vi "QD_git.vi"(6 "Variant in":variant, 7 "Shift Pressed?":bool, 8 "error in (no error)":errorcluster, 10 "QD Combo Box Ref":refnum<vi>, 11 "QD Launch VI Ref":refnum<vi>) -> (0 "error out":errorcluster, 4 "Variant out":variant)   [LabVIEW 2020, in "AJ_QuickDrop_Git.lvlib"]
doc: "Write a 1-2 sentence description of the functionality of your plugin here. Replace the \"$\" below with the character you wish to assign as the default shortcut for this plugin. Do not add any text after the 'Default Shortcut' line below.\n\nDefault Shortcut - [$]"
uses:
  <resource>/dialog/QuickDrop/plugins/AJ_QD_Git/AJ_QuickDrop_Git.lvlib
panel:
  in  "Undo Name":string="Quick Drop Keyboard Shortcut"
  # "Do not change the connector pane of this VI.\n\nSee the block diagram for directions on how to use this template."
  # "Specify the name of the Undo transaction"
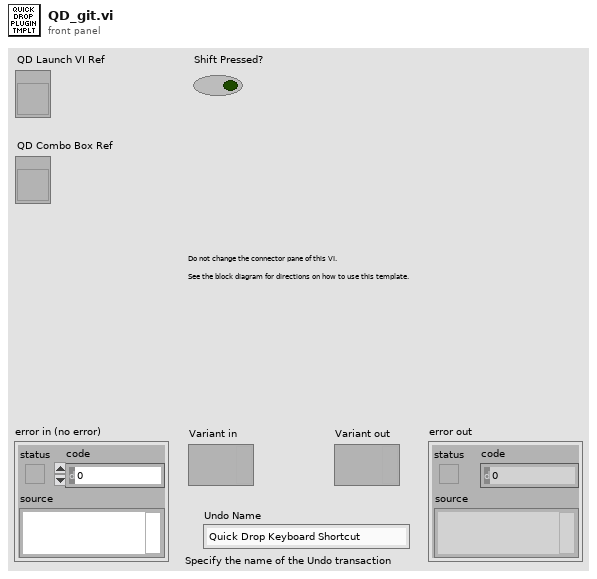
[diagram p1: front panel]
types:
  T1 = enum32{"Invalid", "Standard", "Closed", "Hidden", "Minimized", "Maximized"}
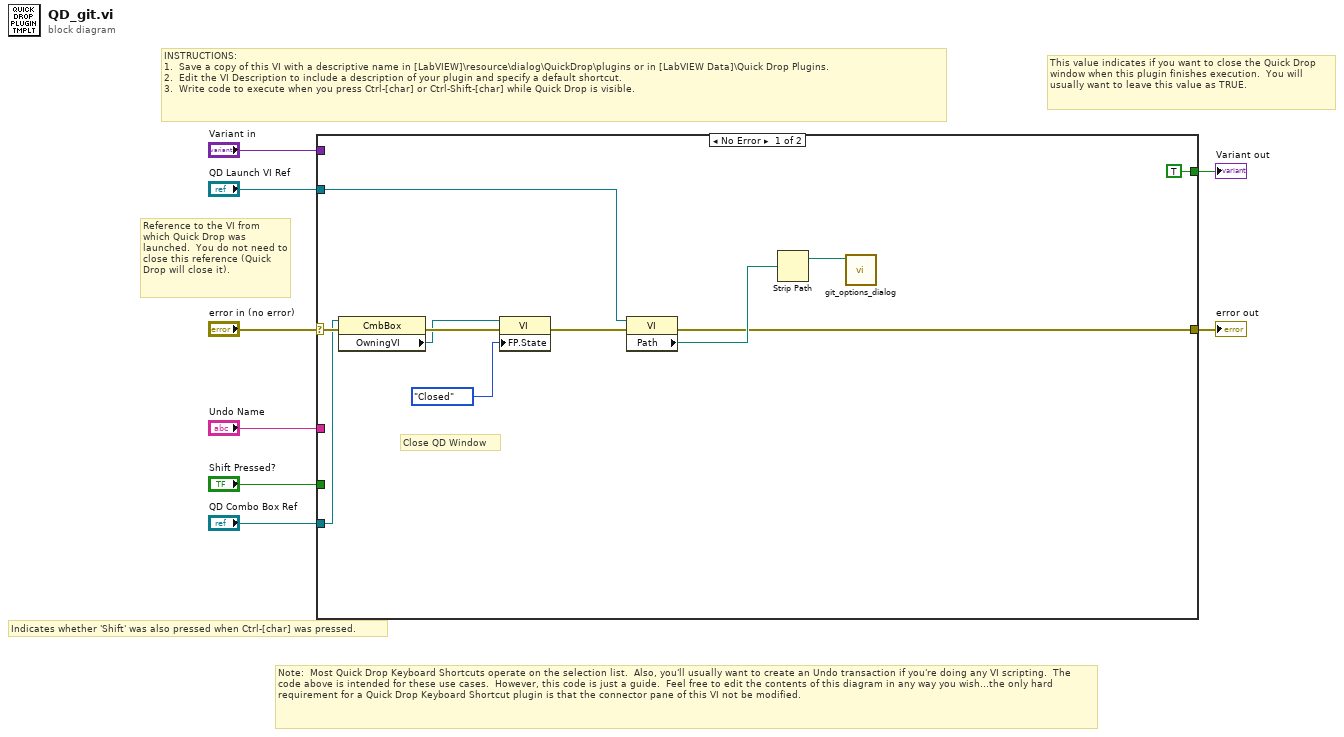
[diagram p0: block diagram]
diagram:
  # "Note:  Most Quick Drop Keyboard Shortcuts operate on the selection list.  Also, you'll usually want to create an Undo transaction if you're doing any VI scripting.  The code above is intended for these use cases.  However, this code is just a guide.  Feel free to edit the contents of this diagram in any way you wish...the only hard requirement for a Quick Drop Keyboard Shortcut plugin is that the connector pane of this VI not be modified."
  # "Indicates whether 'Shift' was also pressed when Ctrl-[char] was pressed."
  # "This value indicates if you want to close the Quick Drop window when this plugin finishes execution.  You will usually want to leave this value as TRUE."
  # "Reference to the VI from which Quick Drop was launched.  You do not need to close this reference (Quick Drop will close it)."
  # "INSTRUCTIONS:\n1.  Save a copy of this VI with a descriptive name in [LabVIEW]\\resource\\dialog\\QuickDrop\\plugins or in [LabVIEW Data]\\Quick Drop Plugins.\n2.  Edit the VI Description to include a description of your plugin and specify a default shortcut. \n3.  Write code to execute when you press Ctrl-[char] or Ctrl-Shift-[char] while Quick Drop is visible."
  n1 = case shown="No Error" "error in (no error)" {
    selector: "error in (no error)" -> [w19 w20]
    tunnel: [w16 w20] -> w7
    tunnel: "QD Launch VI Ref" -> [w18 _]
    tunnel: "Shift Pressed?" -> [_ _]
    tunnel: "QD Combo Box Ref" -> [w12 _]
    tunnel: "Variant in" -> [_ _]
    tunnel: "Undo Name" -> [_ _]
    tunnel: [TRUE _] -> w1
    frame No Error {
      # "Close QD Window"
      n2 = property class="CmbBox"(reference=w12, error in=w19) -> (error out=w13:errorcluster, "OwningVI"=w10:refnum<vi>)  [unwired: 1 out]
      n3 = property class="VI"(reference=w10, error in=w13, "FP.State"=T1."Closed" ("Front Panel Window:State")) -> (error out=w11:errorcluster)  [unwired: 1 out]
      n4 = property class="VI"(reference=w18, error in=w11) -> (error out=w16:errorcluster, "Path"=w17:path)  [unwired: 1 out]
      n5 = Strip Path(path=w17) -> (stripped path=w14:path)  [unwired: 1 out]
      n6 = call <resource>:"git_options_dialog.vi"("Working Dir"=w14) -> ()  [unwired: 11 in]
    }
    frame Error {
    }
  }
  "error out" <- w7
  "Variant out" <- w1
